vi "Start Task.vi"(8 "error in":errorcluster, 11 "NI Analog Output in":refnum<class "NI Analog Output.lvclass">) -> (0 "error out":errorcluster, 3 "NI Analog Output out":refnum<class "NI Analog Output.lvclass">)   [LabVIEW 2023, in "HardwareAbstractionLayer_LVOOP.lvlib" / "NI Analog Output.lvclass"]
doc: "This VI is DAQmx Start the Task"
uses:
  NI Analog Output.lvclass
  NI Analog Output.lvclass/NI Analog Output.ctl
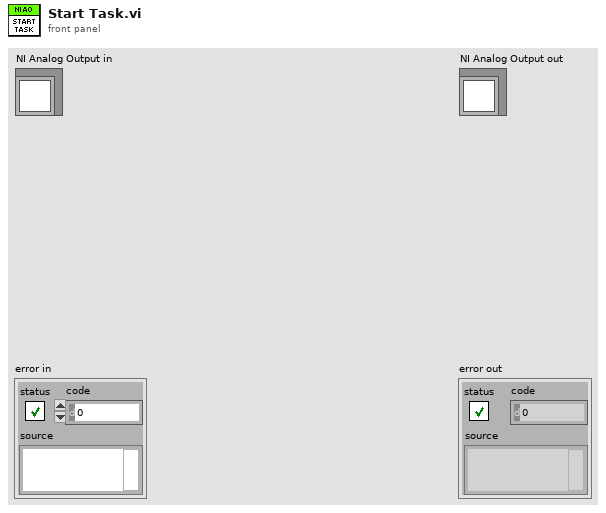
[diagram p1: front panel]
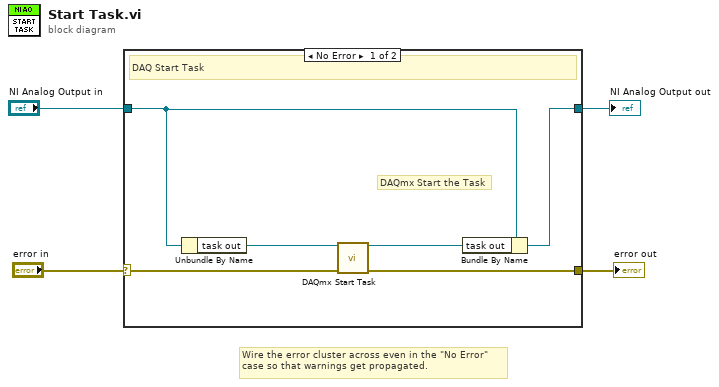
[diagram p0: block diagram]
diagram:
  # "Wire the error cluster across even in the \"No Error\"\ncase so that warnings get propagated."
  n1 = case shown="No Error" "error in" {
    selector: "error in" -> [w10 w12]
    tunnel: [w9 w12] -> w3
    tunnel: [w6 w11] -> w1
    tunnel: "NI Analog Output in" -> [w7 w11]
    frame No Error {
      # "DAQmx Start the Task"
      # "DAQ Start Task"
      n2 = Unbundle By Name(w7) -> ("task out"=w8:refnum<k21>)
      n3 = call <vilib>:"DAQmx Start Task.vi"("task/channels in"=w8, "error in"=w10) -> ("task out"=w5:refnum<k21>, "error out"=w9:errorcluster)  [unwired: 12 in]
      n4 = Bundle By Name(cluster=w7, "task out"=w5) -> (w6:refnum<class "NI Analog Output.lvclass">)
    }
    frame Error {
    }
  }
  "error out" <- w3
  "NI Analog Output out" <- w1
